vi "Generate Output wrapper.vi"(0 "PIDClass string":string, 1 "Input":dbl) -> (2 "PIDClass string out":string, 3 "Output":dbl, 4 "error out":errorcluster)   [LabVIEW 2011]
uses:
  PIDClass.lvclass
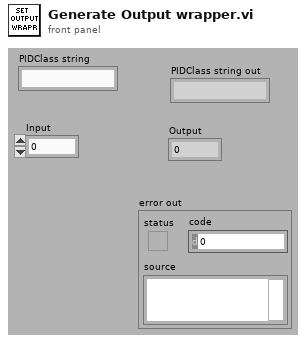
[diagram p1: front panel]
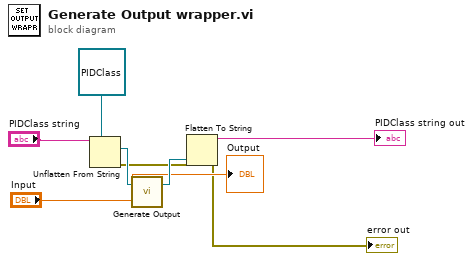
[diagram p0: block diagram]
diagram:
  n1 = Unflatten From String(type=refnum<class "PIDClass.lvclass"> refnum ("PIDClass.lvclass out"), binary string="PIDClass string") -> (value=w7:refnum<class "PIDClass.lvclass">, error out=w2:errorcluster)  [unwired: 1 in, 3 out]
  n2 = call "Generate Output.vi"("Input"="Input", "PIDClass.lvclass"=w7) -> ("Output"=→"Output":dbl, "PIDClass.lvclass out"=w8:refnum<class "PIDClass.lvclass">)
  n3 = Flatten To String(anything=w8, error in (no error)=w2) -> (data string=→"PIDClass string out":string, error out=→"error out":errorcluster)  [unwired: 3 out]
